vi "MTM2_putSample_axialForcesMeasured.vi"(8 "error in (no error)":errorcluster, 11 "axialForcesMeasured_Ctl":T1={"axialForceMeasured[72]"=[0.0, 0.0, 0.0, 0.0, 0.0, 0.0, 0.0, 0.0, 0.0, 0.0, 0.0, 0.0, 0.0, 0.0, 0.0, 0.0, 0.0, 0.0, 0.0, 0.0, 0.0, 0.0, 0.0, 0.0, 0.0, 0.0, 0.0, 0.0, 0.0, 0.0, 0.0, 0.0, 0.0, 0.0, 0.0, 0.0, 0.0, 0.0, 0.0, 0.0, 0.0, 0.0, 0.0, 0.0, 0.0, 0.0, 0.0, 0.0, 0.0, 0.0, 0.0, 0.0, 0.0, 0.0, 0.0, 0.0, 0.0, 0.0, 0.0, 0.0, 0.0, 0.0, 0.0, 0.0, 0.0, 0.0, 0.0, 0.0, 0.0, 0.0, 0.0, 0.0]}) -> (0 "error out":errorcluster, 2 "function return":i32, 3 "axialForcesMeasured_Ctl out":T1)   [LabVIEW 2018, in "SALLV_MTM2.lvlib"]
doc: "int MTM2_shm_putSample_axialForcesMeasuredLV(MTM2_axialForcesMeasuredLV *axialForcesMeasured_Ctl );"
uses:
  SALLV_MTM2.lvlib
  DataTypes/axialForcesMeasured.ctl
  SALLV_MTM2.so
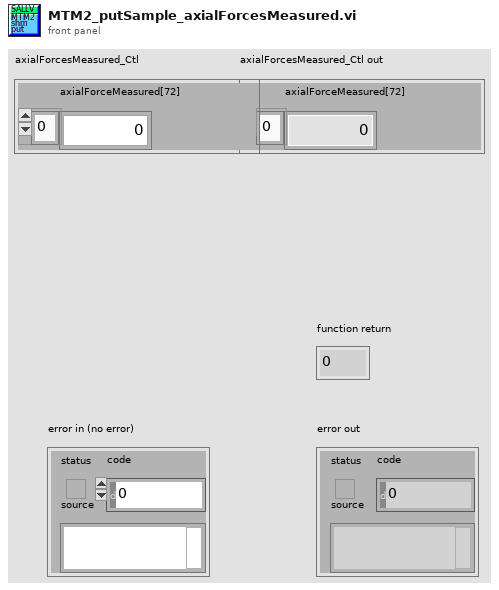
[diagram p1: front panel]
types:
  T1 = typedef "SALLV_MTM2.lvlib/axialForcesMeasured.ctl" = cluster{"axialForceMeasured[72]":dbl[]}
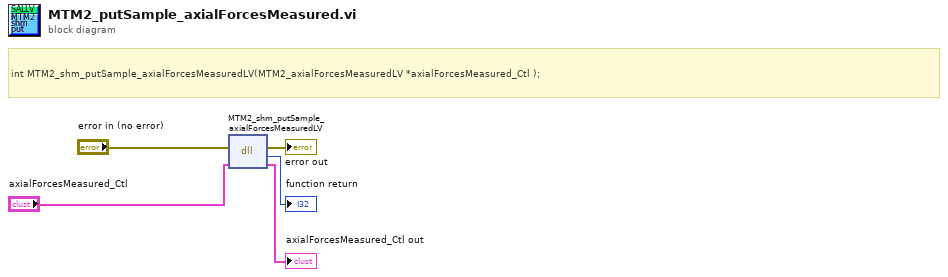
[diagram p0: block diagram]
diagram:
  # "int MTM2_shm_putSample_axialForcesMeasuredLV(MTM2_axialForcesMeasuredLV *axialForcesMeasured_Ctl );"
  n1 = dll-call lib="home/ttsai/Document/salApiMTM2/SALLV_MTM2/SALLV_MTM2.*" fn="MTM2_shm_putSample_axialForcesMeasuredLV"(error in="error in (no error)", "axialForcesMeasured_Ctl"="axialForcesMeasured_Ctl") -> (error out=→"error out":errorcluster, →"function return":i32, "axialForcesMeasured_Ctl"=→"axialForcesMeasured_Ctl out":T1)  [unwired: 2 in, 1 out]
